vi "Untitled 1.vi"() -> ()   [LabVIEW 2014]
panel:
  out "error out 2":errorcluster
  out "data out 2":string
  out "Numeric 2":i32
  out "error out":errorcluster
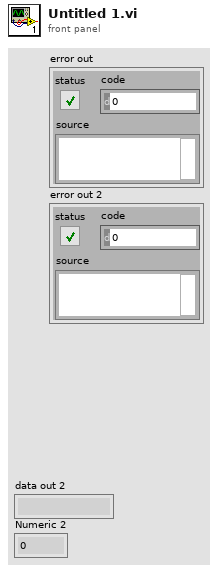
[diagram p1: front panel]
types:
  T1 = enum16{"Standard", "Buffered", "CRLF", "Immediate"}
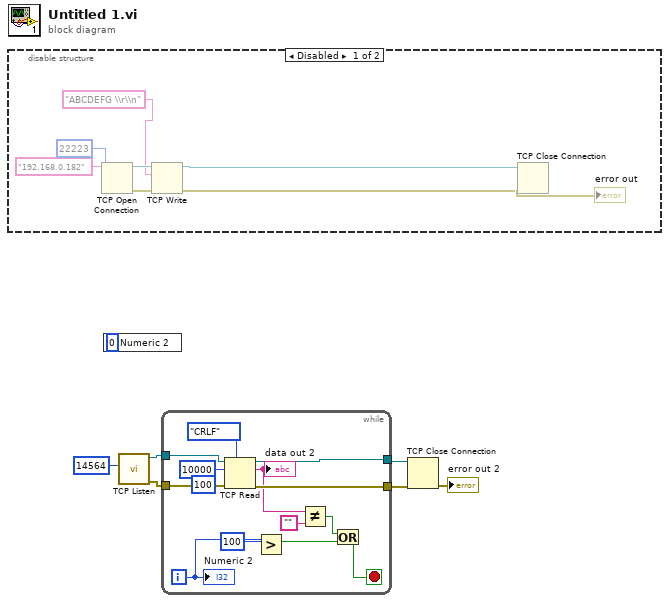
[diagram p0: block diagram]
diagram:
  n1 = disable-structure shown="Disabled" {
    frame Disabled {
      n2 = TCP Open Connection(address="192.168.0.182", remote port or service name=u16 22223) -> (connection ID=w12:refnum<k5>, error out=w13:errorcluster)  [unwired: 3 in]
      n3 = TCP Write(connection ID=w12, data in="ABCDEFG \\r\\n", error in (no error)=w13) -> (connection ID out=w9:refnum<k5>, error out=w8:errorcluster)  [unwired: 1 in, 1 out]
      n4 = TCP Close Connection(connection ID=w9, error in (no error)=w8) -> (error out=→"error out":errorcluster)  [unwired: 1 in, 1 out]
    }
    frame Enabled {
    }
  }
  n5 = local write "Numeric 2"(0) -> ()
  n6 = call <vilib>:"TCP Listen.vi"("port"=u16 14564) -> ("error out"=w5:errorcluster, "connection ID"=w6:refnum<k5>)  [unwired: 6 in, 3 out]
  n7 = while {
    tunnel: [w29] -> w4
    tunnel: [w28] -> w3
    tunnel: w6 -> [w18]
    tunnel: w5 -> [w17]
    i -> [w23]
    stop <- w21 stop-if-true
    n8 = TCP Read(connection ID=w18, bytes to read=10000, error in (no error)=w17, 7:T1."CRLF" ("mode (standard)"), 9:100 ("timeout ms (25000)")) -> (connection ID out=w29:refnum<k5>, data out=w25:string, error out=w28:errorcluster)
    "data out 2" <- w25
    n9 = Greater?(x=w23, y=100) -> (0:w20:bool)
    n10 = Not Equal?(x=w25, y="") -> (x != y?=w19:bool)
    n11 = Or(x=w19, y=w20) -> (x .or. y?=w21:bool)
    "Numeric 2" <- w23
  }
  n12 = TCP Close Connection(connection ID=w4, error in (no error)=w3) -> (error out=→"error out 2":errorcluster)  [unwired: 1 in, 1 out]
